vi "Write Server-URL.vi"(8 "error in (no error)":errorcluster, 10 "Server-URL":string, 11 "ByteGSWebAPI-V0 in":refnum<class "ByteGSWebAPI-V0.lvclass">) -> (0 "error out":errorcluster, 3 "ByteGSWebAPI-V0 out":refnum<class "ByteGSWebAPI-V0.lvclass">)   [LabVIEW 2019, in "ByteGSWebAPI.lvlib" / "ByteGSWebAPI-V0.lvclass"]
uses:
  ByteGSWebAPI-V0.lvclass
  ByteGSWebAPI-V0.lvclass/ByteGSWebAPI-V0.ctl
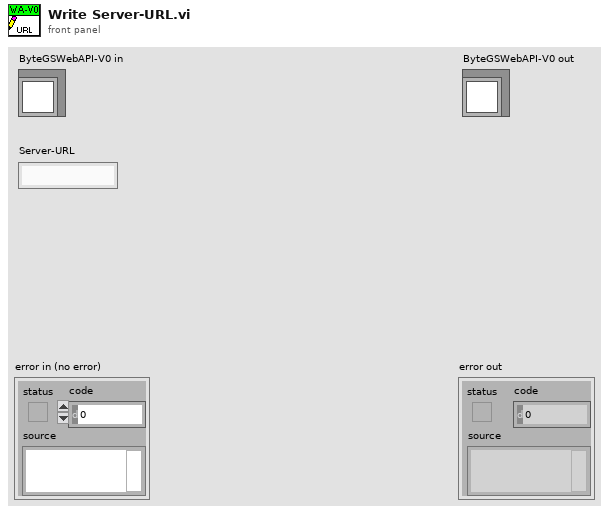
[diagram p1: front panel]
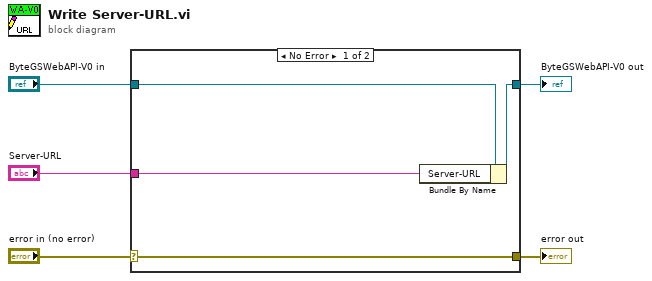
[diagram p0: block diagram]
diagram:
  n1 = case shown="No Error" "error in (no error)" {
    selector: "error in (no error)" -> [w9 w10]
    tunnel: [w9 w10] -> w4
    tunnel: [w7 w11] -> w2
    tunnel: "ByteGSWebAPI-V0 in" -> [w8 w11]
    tunnel: "Server-URL" -> [w6 _]
    frame No Error {
      n2 = Bundle By Name(cluster=w8, "Server-URL"=w6) -> (w7:refnum<class "ByteGSWebAPI-V0.lvclass">)
    }
    frame Error {
    }
  }
  "error out" <- w4
  "ByteGSWebAPI-V0 out" <- w2
